vi "Start.vi"(8 "error in (no error)":errorcluster, 10 "Message in":refnum<class "StartMessage.lvclass">, 11 "Galvo in":refnum<class "ImagingModeSPIM.lvclass">) -> (0 "error out":errorcluster, 3 "Galvo out":refnum<class "ImagingModeSPIM.lvclass">)   [LabVIEW 2012, in "ImagingModeSPIM.lvclass"]
doc: "This member function is called when the statemachine in the run.vi receives an 'start' command. It relays the message to all observers of the component.\n\nOverride this member function in your derived class if you need additional start functionality (but don't forget to call the parent method)."
uses:
  ImagingModeSPIM.lvclass
  <vilib>/Distrio/Murmex/StartMessage/StartMessage.lvclass
  <vilib>/Distrio/Murmex/Murmex/Murmex.lvclass
  <vilib>/Distrio/Murmex/StartMessage/run mode enum.ctl
  ImagingModeSPIM.lvclass/ImagingModeSPIM.ctl
  <vilib>/Distrio/Murmex/StartMessage/Get run mode.vi
  <vilib>/Distrio/Murmex/ProceedMessage/ProceedMessage.lvclass
panel:
  # "This member function is called when the statemachine in the run.vi receives an 'start' command. It relays the message to all observers of the component.\n\nOverride this member function in your derived class if you need additional start functionality (but don't forget to call the parent method)."
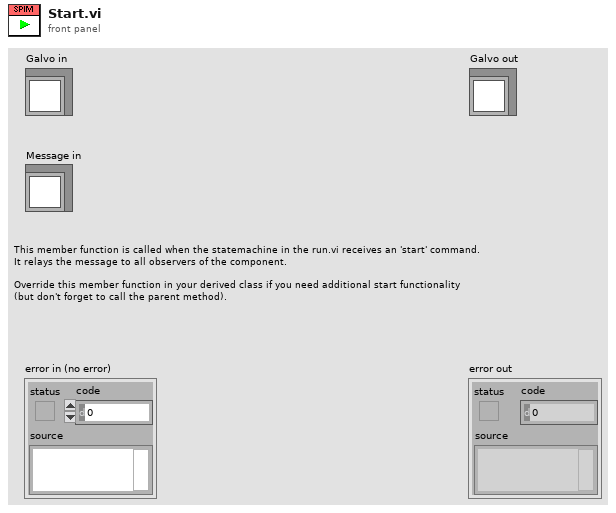
[diagram p1: front panel]
types:
  T1 = typedef "Murmex.lvlib/StartMessage.lvclass/run mode enum.ctl" = enum16{"infinite", "finite"}
  T2 = enum8{"Enabled", "Disabled", "Disabled and Grayed Out"}
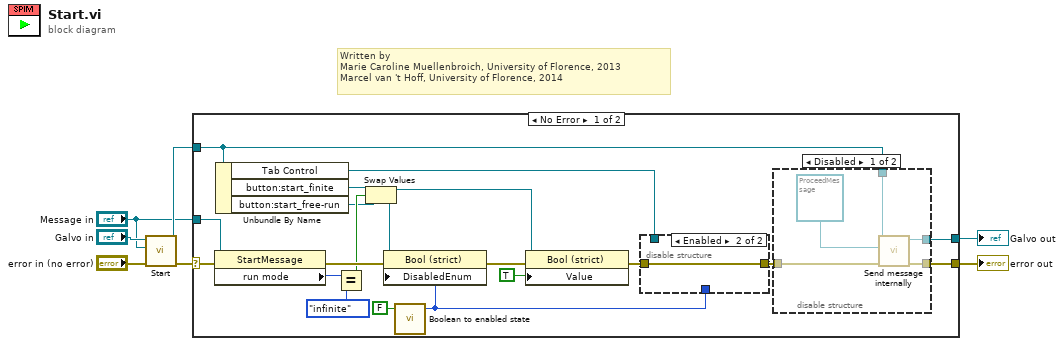
[diagram p0: block diagram]
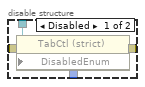
[diagram p3: hidden frame]
diagram:
  # "Written by \nMarie Caroline Muellenbroich, University of Florence, 2013 \nMarcel van 't Hoff, University of Florence, 2014"
  n1 = call-parent "Start.vi"("error in (no error)"="error in (no error)", "Message in"="Message in", "Murmex in"="Galvo in") -> ("error out"=w4:errorcluster, "Murmex out"=w5:refnum<class "ImagingModeSPIM.lvclass">)  [unwired: 7 in]
  n2 = case shown="No Error" w4 {
    selector: w4 -> [w24 w41]
    tunnel: w5 -> [w23 w40]
    tunnel: [w27 w41] -> w3
    tunnel: [w26 w40] -> w2
    tunnel: "Message in" -> [w25 _]
    frame No Error {
      n3 = property class="StartMessage"(reference=w25, error in=w24) -> (error out=w19:errorcluster, "run mode"=w22:T1)  [unwired: 1 out]
      n4 = Unbundle By Name(w23) -> ("Tab Control"=w18:refnum<vi>, "button:start_finite"=w14:refnum<vi>, "button:start_free-run"=w13:refnum<vi>)
      n5 = Equal?(x=w22, y=run_mode_enum."infinite" ("run mode")) -> (x = y?=w15:bool)
      n6 = Swap Values(12:w14, 13:w15, 14:w13) -> (1:w9:refnum<vi>, 3:w8:refnum<vi>)
      n7 = call <vilib>:"Boolean to enabled state.vi"("boolean in"=FALSE) -> ("enabled status out"=w17:T2)  [unwired: 4 in]
      n8 = property class="Bool (strict)"(reference=w8, error in=w19, "DisabledEnum"=w17) -> (error out=w11:errorcluster)  [unwired: 1 out]
      n9 = property class="Bool (strict)"(reference=w9, error in=w11, "Value"=TRUE) -> (error out=w10:errorcluster)  [unwired: 1 out]
      n10 = disable-structure shown="Enabled" {
        disable-tunnel: w18 -> [w38 _]
        disable-tunnel: w17 -> [w37 _]
        disable-tunnel: [w36 w39] -> w16
        disable-tunnel: w10 -> [w35 w39]
        frame Disabled {
          n11 = property class="TabCtl (strict)"(reference=w38, error in=w35, "DisabledEnum"=w37) -> (error out=w36:errorcluster)  [unwired: 1 out]
        }
        frame Enabled {
        }
      }
      n12 = disable-structure shown="Disabled" {
        disable-tunnel: [w32 w33] -> w27
        disable-tunnel: [w31 w34] -> w26
        disable-tunnel: w23 -> [w30 w34]
        disable-tunnel: w16 -> [w29 w33]
        frame Disabled {
          n13 = call <vilib>:"Send message internally.vi"("error in (no error)"=w29, "Message"=refnum<class "ProceedMessage.lvclass"> refnum ("Murmex.lvlib:ProceedMessage"), "Murmex in"=w30) -> ("error out"=w32:errorcluster, "Murmex out"=w31:refnum<class "ImagingModeSPIM.lvclass">)  [unwired: 7 in]
        }
        frame Enabled {
        }
      }
    }
    frame Error {
    }
  }
  "error out" <- w3
  "Galvo out" <- w2
